vi "读欧姆龙PLC.vi"(1 "写入缓冲区":string, 2 "簇":T1={"VISA resource name"="", "baud rate (9600)"=9600, "data bits (8)"=8, "parity (0:none)"=enum."None", "stop bits (10: 1 bit)"=10, "timeout (10sec)"=10000} {"stop bits (10: 1 bit)" items=["1.0"=10, "1.5"=15, "2.0"=20]}) -> (0 "读取缓冲区":string)   [LabVIEW 2012]
uses:
  <vilib>/Instr/_visa.llb/VISA Configure Serial Port (Instr).vi
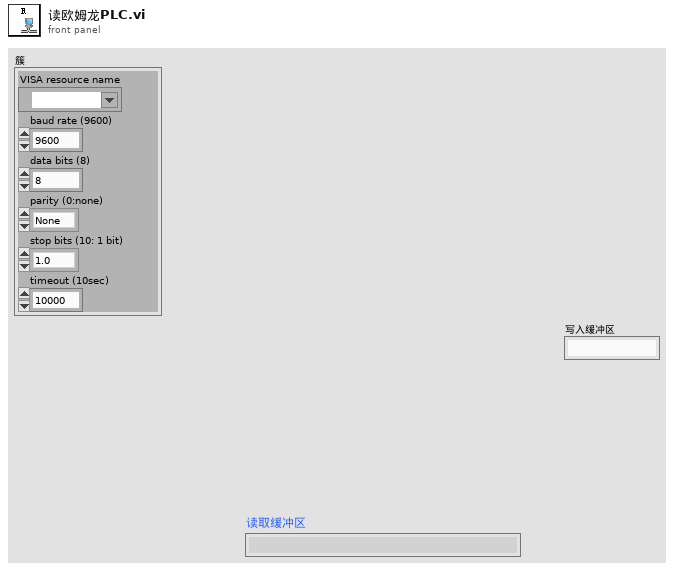
[diagram p1: front panel]
types:
  T1 = cluster{"VISA resource name":refnum<visa-resource-name>, "baud rate (9600)":u32, "data bits (8)":u16, "parity (0:none)":enum16{"None", "Odd", "Even", "Mark", "Space"}, "stop bits (10: 1 bit)":u16, "timeout (10sec)":u32}
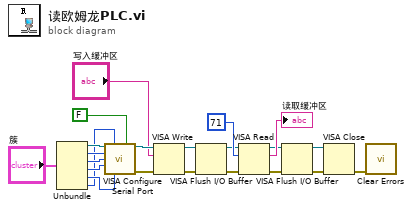
[diagram p0: block diagram]
diagram:
  n1 = Unbundle("簇") -> ("VISA resource name"=w6:refnum<visa-resource-name>, "baud rate (9600)"=w5:u32, "data bits (8)"=w4:u16, "parity (0:none)"=w3:enum16{"None", "Odd", "Even", "Mark", "Space"}, "stop bits (10: 1 bit)"=w2:u16, "timeout (10sec)"=w1:u32)
  n2 = call-poly "VISA Configure Serial Port"("VISA resource name"=w6, "timeout (10sec)"=w1, "Enable Termination\nChar (T)"=FALSE ("Enable Termination\nChar (T)"), "baud rate (9600)"=w5, "data bits (8)"=w4, "parity (0:none)"=w3, "stop bits (10: 1 bit)"=w2) -> ("VISA resource name out"=w19:refnum<visa-resource-name>, "error out"=w20:errorcluster)  [unwired: 7 in]
  n3 = VISA Write(VISA resource name=w19, write buffer="写入缓冲区", error in (no error)=w20) -> (VISA resource name out=w21:refnum<visa-resource-name>, error out=w22:errorcluster)  [unwired: 1 out]
  n4 = VISA Flush I/O Buffer(VISA resource name=w21, error in (no error)=w22) -> (VISA resource name out=w14:refnum<visa-resource-name>, error out=w13:errorcluster)  [unwired: 1 in]
  n5 = VISA Read(VISA resource name=w14, byte count=u32 71 ("字节总数"), error in (no error)=w13) -> (VISA resource name out=w12:refnum<visa-resource-name>, read buffer=→"读取缓冲区":string, error out=w11:errorcluster)  [unwired: 1 out]
  n6 = VISA Flush I/O Buffer(VISA resource name=w12, error in (no error)=w11) -> (VISA resource name out=w10:refnum<visa-resource-name>, error out=w9:errorcluster)  [unwired: 1 in]
  n7 = VISA Close(VISA resource name=w10, error in (no error)=w9) -> (error out=w8:errorcluster)
  n8 = call <vilib>:"Clear Errors.vi"("error in (no error)"=w8) -> ()  [unwired: 6 in, 1 out]
